vi "SET_UserLayers.vi"(8 "error in (no error)":errorcluster, 10 "Layers":refnum<class "Layer.lvclass">[](array[class]), 11 "Icon.lvclass in":refnum<class "Icon.lvclass">) -> (0 "error out":errorcluster, 3 "Icon.lvclass out":refnum<class "Icon.lvclass">)   [LabVIEW 2020, in "Icon.lvclass"]
doc: "Sets all User Layers."
uses:
  Icon.lvclass
  Layer/Layer.lvclass
  Icon.lvclass/Icon.ctl
  lv_icon.lvlib
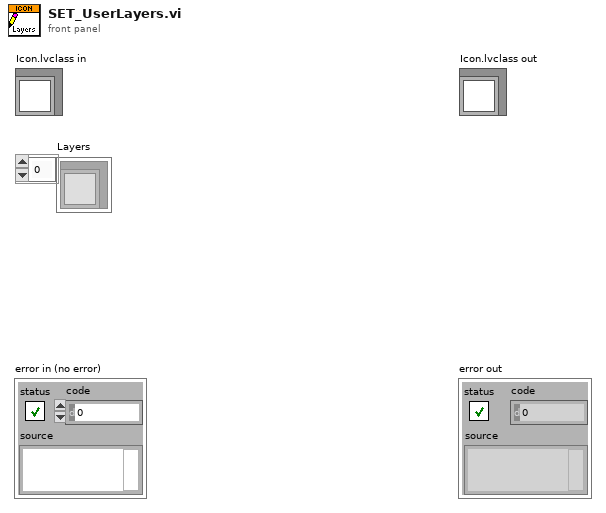
[diagram p1: front panel]
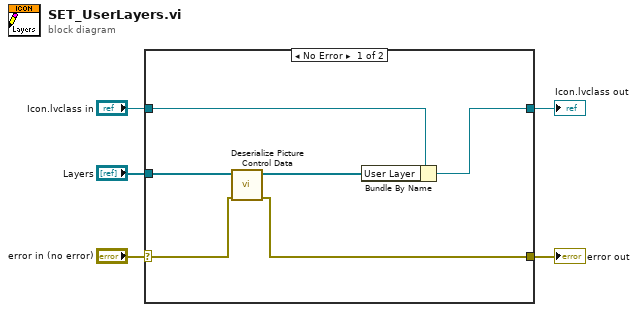
[diagram p0: block diagram]
diagram:
  n1 = case shown="No Error" "error in (no error)" {
    selector: "error in (no error)" -> [w8 w12]
    tunnel: [w6 w12] -> w4
    tunnel: [w10 w13] -> w2
    tunnel: "Icon.lvclass in" -> [w11 w13]
    tunnel: "Layers" -> [w9 _]
    frame No Error {
      n2 = call "Deserialize Picture Control Data.vi"("error in (no error)"=w8, "Layers in"=w9) -> ("error out"=w6:errorcluster, "Layers out"=w7:refnum<class "Layer.lvclass">[])  [unwired: 8 out]
      n3 = Bundle By Name(cluster=w11, "User Layer"=w7) -> (w10:refnum<class "Icon.lvclass">)
    }
    frame Error {
    }
  }
  "error out" <- w4
  "Icon.lvclass out" <- w2
